vi "Get Wavelength.vi"(1 "Channel":i32=1) -> (0 "Wavelength (nm)":dbl)   [LabVIEW 2020]
uses:
  Laser Parameters.vi
panel:
  out "body":string
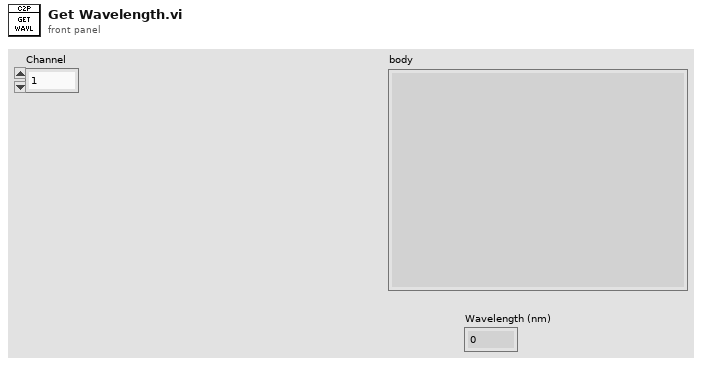
[diagram p1: front panel]
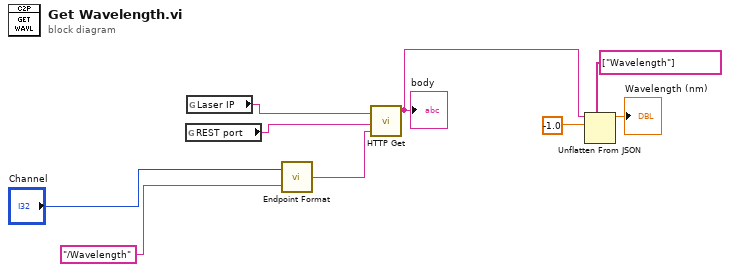
[diagram p0: block diagram]
diagram:
  n1 = global read "Laser Parameters.vi" "REST port"() -> (w8:string)
  n2 = global read "Laser Parameters.vi" "Laser IP"() -> (w9:string)
  n3 = call "Endpoint Format.vi"("Endpoint"="/Wavelength", "Channel"="Channel") -> ("Endpoint URL"=w5:string)
  n4 = call "HTTP Get.vi"("Endpoint"=w5, "Port"=w8, "IP Address"=w9) -> ("body"=w1:string)  [unwired: 1 in, 1 out]
  "body" <- w1
  n5 = Unflatten From JSON(path=string[] ["Wavelength"], JSON string=w1, type and defaults=-1.0) -> (value=→"Wavelength (nm)":dbl)  [unwired: 4 in, 1 out]
